vi "getIPConfig.vi"(8 "error in (no error)":errorcluster, 9 "Data":u8[](array[numeric]), 10 "Device":i32, 11 "SEDSpectrometer in":refnum<class "FiberSpectrograph.lvclass">) -> (0 "error out":errorcluster, 1 "Data":u8[](array[numeric]), 2 "Output Value":i32, 3 "SEDSpectrometer out":refnum<class "FiberSpectrograph.lvclass">)   [LabVIEW 2016, in "FiberSpectrograph.lvclass"]
uses:
  FiberSpectrograph.lvclass
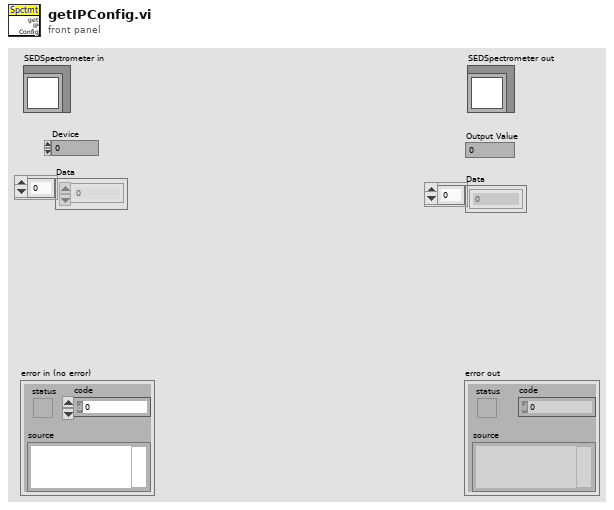
[diagram p1: front panel]
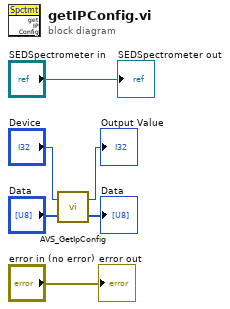
[diagram p0: block diagram]
diagram:
  n1 = call "AVS_GetIpConfig.vi"("a_Data"="Data", "a_hDevice"="Device") -> ("a_Data"=→"Data":u8[], "Output Value"=→"Output Value":i32)
  "error out" <- "error in (no error)"
  "SEDSpectrometer out" <- "SEDSpectrometer in"
